vi "Host - INS DVL Data (SubVI).vi"(11 "INS DVL Data":string) -> (3 "INS DVL Data":dbl[](array[numeric]))   [LabVIEW 2021]
panel:
  out "TIME":string
  out "INS Repeater Status":dbl format="%#_15g"
  out "INS System Status LSB":dbl
  out "INS System Status MSB":dbl
  out "INS Algo Status LSB":dbl format="%#_6f"
  out "INS Algo Status MSB":dbl
  out "East speed std":dbl
  out "North speed std":dbl
  out "Vertical speed std":dbl
  out "Longitude std":dbl
  out "Latitude std":dbl
  out "Altitude std":dbl
  out "Roll std":dbl
  out "Heading std":dbl
  out "Pitch std":dbl
  out "SWAY":dbl
  out "SURGE":dbl
  out "HEAVE":dbl
  out "Altitude GPS":dbl format="%#.3f"
  out "GPS Quality Indicator":dbl
  out "GPS Time":dbl format="%#.3f"
  out "Lat GPS":dbl format="%#.8f"
  out "Long GPS":dbl format="%#.8f"
  out "Depth":dbl format="%#.10f"
  out "Depth Time":dbl
  out "East UTM Pos":dbl format="%#.3f"
  out "ALTITUDE":dbl
  out "LAT UTM Zone":string
  out "LONG UTM Zone":string
  out "North UTM Pos":dbl format="%#.3f"
  out "North speed":dbl
  out "East speed":dbl
  out "UP speed":dbl
  out "Longitude":dbl
  out "Latitude":dbl
  out "Altitude":dbl
  out "ROLL":dbl format="%#.10f"
  out "PITCH":dbl
  out "array 7":string[](array[string])
  out "HEADING__2":dbl
  out "array 6":string[](array[string])
  out "HEADING_1":dbl
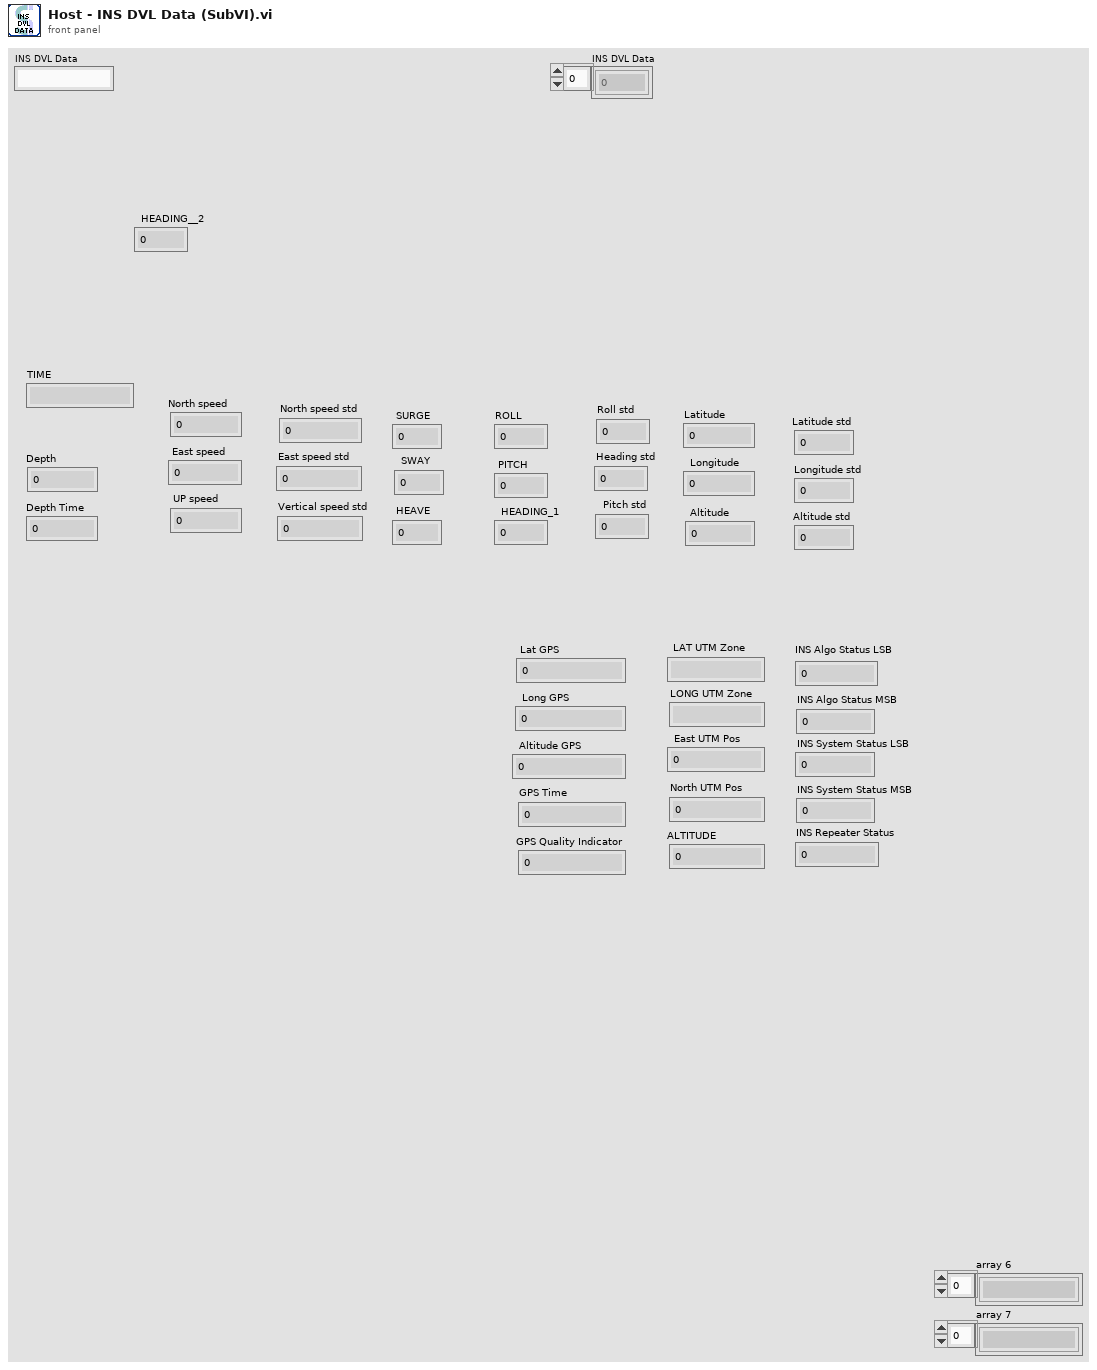
[diagram p1: front panel]
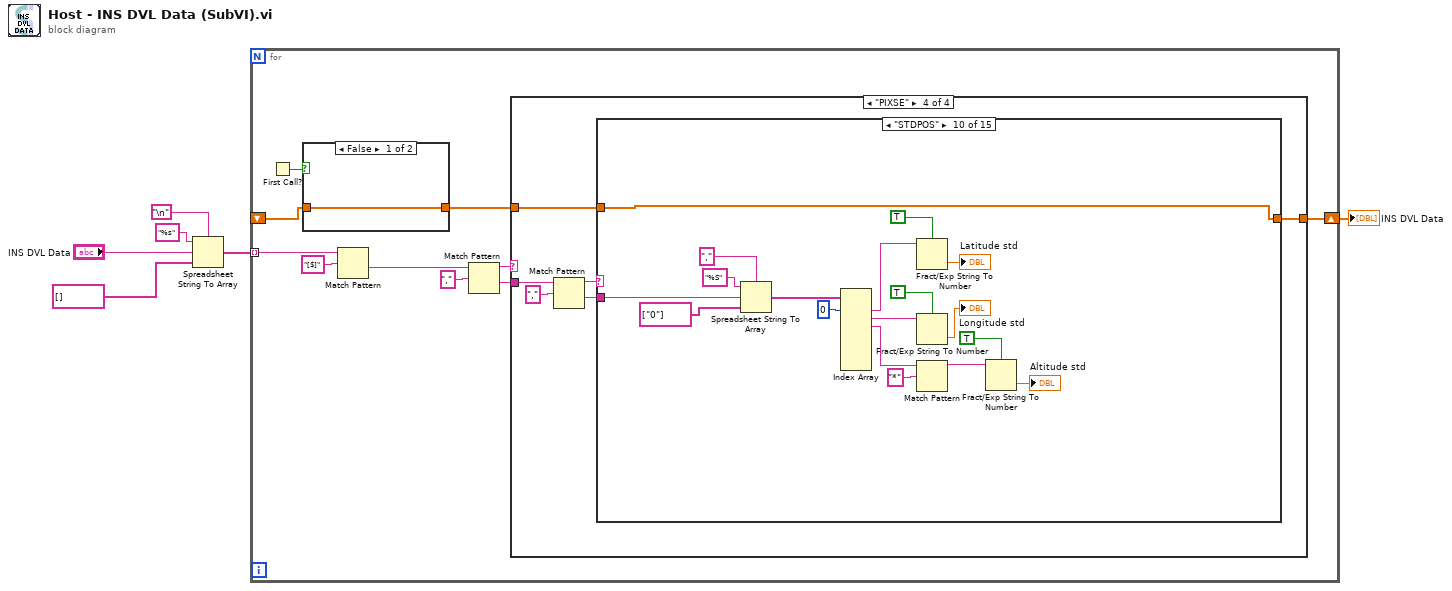
[diagram p0: block diagram]
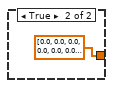
[diagram p2: hidden frame]
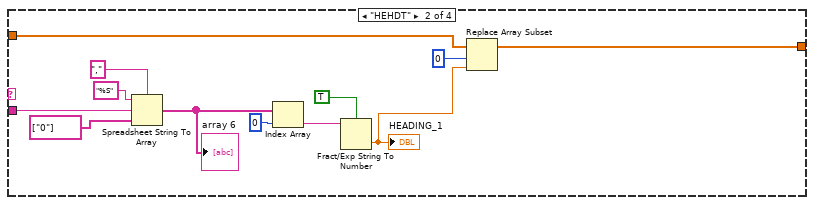
[diagram p4: hidden frame]
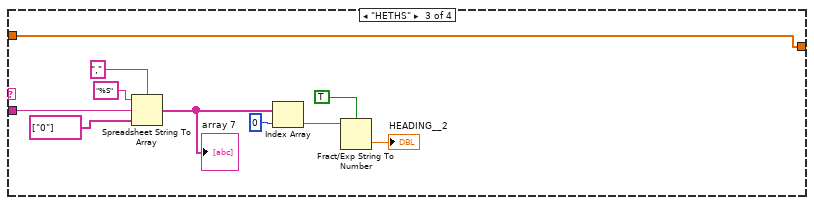
[diagram p5: hidden frame]
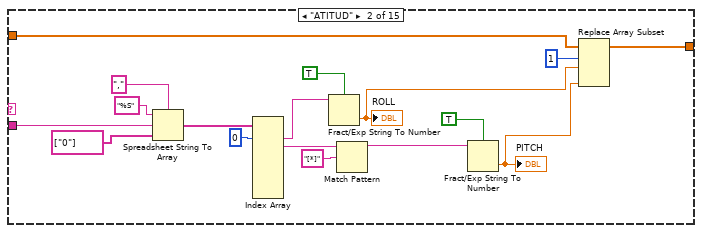
[diagram p7: hidden frame]
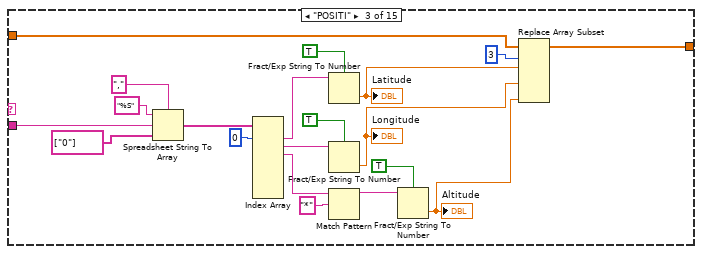
[diagram p8: hidden frame]
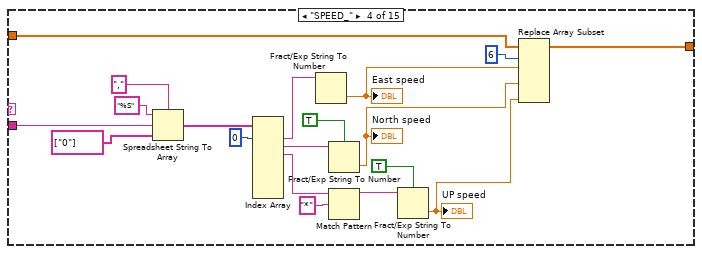
[diagram p9: hidden frame]
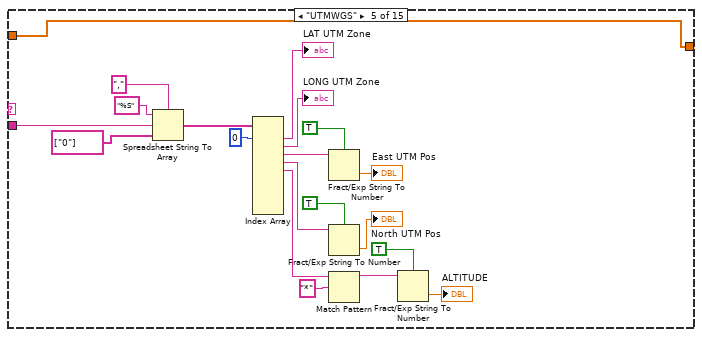
[diagram p10: hidden frame]
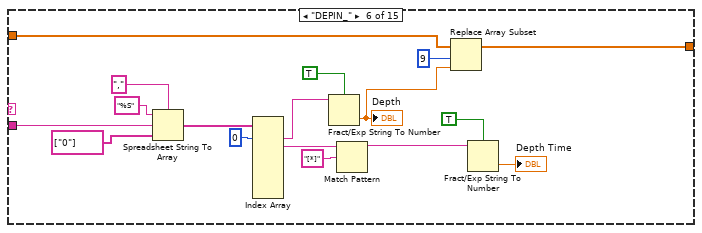
[diagram p11: hidden frame]
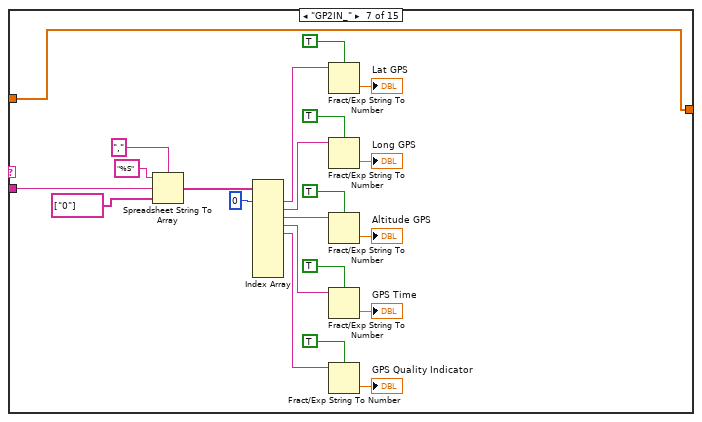
[diagram p12: hidden frame]
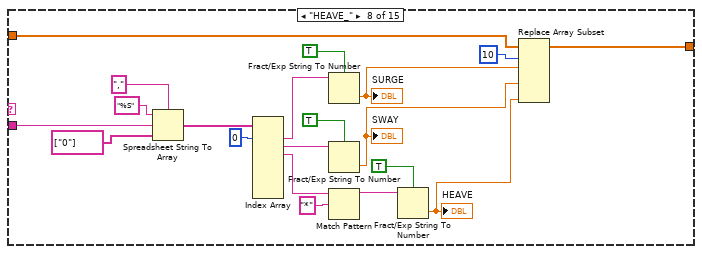
[diagram p13: hidden frame]
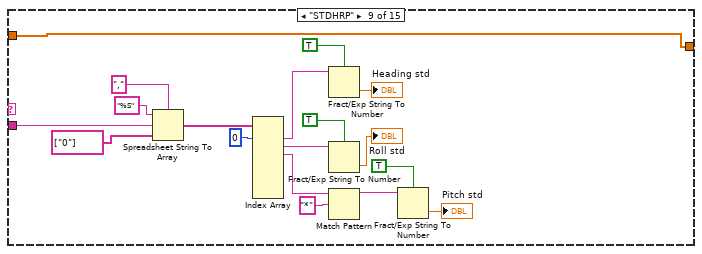
[diagram p14: hidden frame]
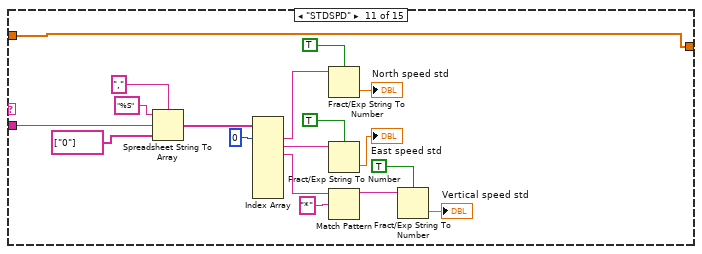
[diagram p15: hidden frame]
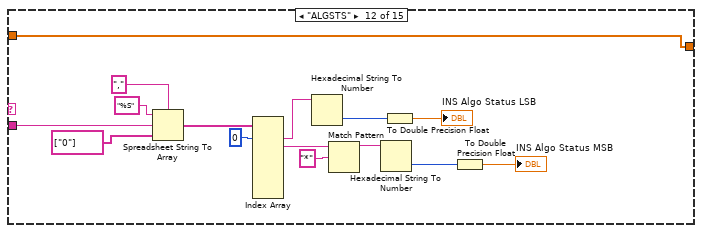
[diagram p16: hidden frame]
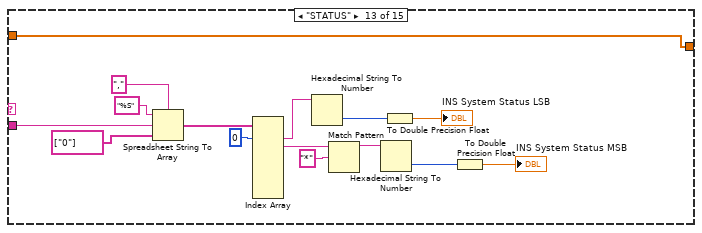
[diagram p17: hidden frame]
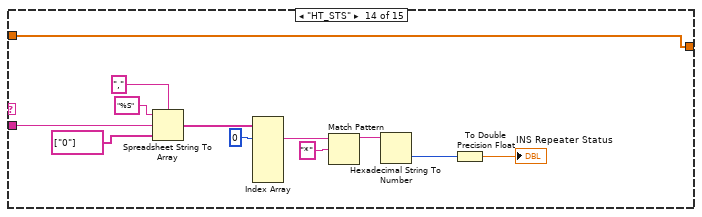
[diagram p18: hidden frame]
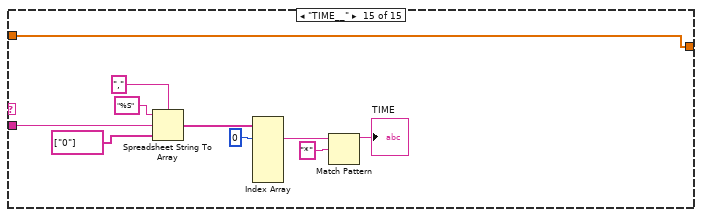
[diagram p19: hidden frame]
diagram:
  n1 = Spreadsheet String To Array(delimiter (Tab)="\n", format string="%s", spreadsheet string="INS DVL Data", array type (2D Dbl)=string[] []) -> (array=w3:string[])
  n2 = for {
    tunnel: w3 -> [w11] mode=indexing
    shift-right: [w10] -> w1
    shift-left: _ -> [w7]
    n3 = First Call?() -> (First Call?: T/F=w9:bool)
    n4 = case shown="False" w9 {
      tunnel: [w17 dbl[] [0.0, 0.0, 0.0, 0.0, 0.0, 0.0, 0.0, 0.0, 0.0, 0.0, 0.0, 0.0, 0.0]] -> w8
      tunnel: w7 -> [w17 _]
      frame False {
      }
      frame True {
      }
    }
    n5 = Match Pattern(string=w11, regular expression="[$]") -> (after substring=w15:string)  [unwired: 1 in, 3 out]
    n6 = Match Pattern(string=w15, regular expression=",") -> (before substring=w13:string, after substring=w12:string)  [unwired: 1 in, 2 out]
    n7 = case shown="\"PIXSE\"" w13 {
      tunnel: w12 -> [_ w28 w38 w47]
      tunnel: w8 -> [w19 w23 w32 w43]
      tunnel: [w19 w22 w32 w42] -> w10
      frame "False", Default {
      }
      frame "HEHDT" {
        n8 = Spreadsheet String To Array(delimiter (Tab)=",", format string="%S", spreadsheet string=w28, array type (2D Dbl)=string[] ["0"]) -> (array=w26:string[])
        "array 6" <- w26
        n9 = Index Array(array=w26, index=0) -> (element=w24:string)
        n10 = Fract/Exp String To Number(use system decimal point (T)=TRUE, string=w24) -> (number=w20:dbl)  [unwired: 2 in, 1 out]
        "HEADING_1" <- w20
        n11 = Replace Array Subset(array=w23, new element=w20, index=0) -> (w22:dbl[])
      }
      frame "HETHS" {
        n12 = Spreadsheet String To Array(delimiter (Tab)=",", format string="%S", spreadsheet string=w38, array type (2D Dbl)=string[] ["0"]) -> (array=w34:string[])
        "array 7" <- w34
        n13 = Index Array(array=w34, index=0) -> (element=w35:string)
        n14 = Fract/Exp String To Number(use system decimal point (T)=TRUE, string=w35) -> (number=→"HEADING__2":dbl)  [unwired: 2 in, 1 out]
      }
      frame "PIXSE" {
        n15 = Match Pattern(string=w47, regular expression=",") -> (before substring=w45:string, after substring=w44:string)  [unwired: 1 in, 2 out]
        n16 = case shown="\"STDPOS\"" w45 {
          tunnel: w44 -> [_ w62 w82 w101 w121 w129 w150 w183 w198 w204 w234 w249 w264 w276 w286]
          tunnel: w43 -> [w48 w53 w70 w90 w105 w127 w142 w168 w184 w202 w220 w238 w253 w268 w280]
          tunnel: [w48 w52 w71 w91 w105 w128 w142 w169 w184 w202 w220 w238 w253 w268 w280] -> w42
          frame "False", Default {
          }
          frame "ATITUD" {
            n17 = Spreadsheet String To Array(delimiter (Tab)=",", format string="%S", spreadsheet string=w62, array type (2D Dbl)=string[] ["0"]) -> (array=w61:string[])
            n18 = Index Array(array=w61, index #1=0 ("index")) -> (element #1=w57:string, element #2=w58:string)  [unwired: 7 in, 6 out]
            n19 = Fract/Exp String To Number(use system decimal point (T)=TRUE, string=w57) -> (number=w50:dbl)  [unwired: 2 in, 1 out]
            "ROLL" <- w50
            n20 = Match Pattern(string=w58, regular expression="[*]") -> (before substring=w55:string)  [unwired: 1 in, 3 out]
            n21 = Fract/Exp String To Number(use system decimal point (T)=TRUE, string=w55) -> (number=w49:dbl)  [unwired: 2 in, 1 out]
            "PITCH" <- w49
            n22 = Replace Array Subset(array=w53, new element #1=w50, index #1=1 ("index"), new element #2=w49) -> (w52:dbl[])  [unwired: 1 in]
          }
          frame "POSITI" {
            n23 = Spreadsheet String To Array(delimiter (Tab)=",", format string="%S", spreadsheet string=w82, array type (2D Dbl)=string[] ["0"]) -> (array=w79:string[])
            n24 = Index Array(array=w79, index #1=0 ("index")) -> (element #1=w81:string, element #2=w72:string, element #3=w74:string)  [unwired: 7 in, 5 out]
            n25 = Fract/Exp String To Number(use system decimal point (T)=TRUE, string=w81) -> (number=w68:dbl)  [unwired: 2 in, 1 out]
            "Latitude" <- w68
            n26 = Fract/Exp String To Number(use system decimal point (T)=TRUE, string=w72) -> (number=w67:dbl)  [unwired: 2 in, 1 out]
            "Longitude" <- w67
            n27 = Match Pattern(string=w74, regular expression="*") -> (before substring=w76:string)  [unwired: 1 in, 3 out]
            n28 = Fract/Exp String To Number(use system decimal point (T)=TRUE, string=w76) -> (number=w66:dbl)  [unwired: 2 in, 1 out]
            "Altitude" <- w66
            n29 = Replace Array Subset(array=w70, new element #1=w68, index #1=3 ("index"), new element #2=w67, new element #3=w66) -> (w71:dbl[])  [unwired: 2 in]
          }
          frame "SPEED_" {
            n30 = Spreadsheet String To Array(delimiter (Tab)=",", format string="%S", spreadsheet string=w101, array type (2D Dbl)=string[] ["0"]) -> (array=w92:string[])
            n31 = Index Array(array=w92, index #1=0 ("index")) -> (element #1=w100:string, element #2=w93:string, element #3=w95:string)  [unwired: 7 in, 5 out]
            n32 = Fract/Exp String To Number(string=w100) -> (number=w88:dbl)  [unwired: 3 in, 1 out]
            "East speed" <- w88
            n33 = Fract/Exp String To Number(use system decimal point (T)=TRUE, string=w93) -> (number=w87:dbl)  [unwired: 2 in, 1 out]
            "North speed" <- w87
            n34 = Match Pattern(string=w95, regular expression="*") -> (before substring=w97:string)  [unwired: 1 in, 3 out]
            n35 = Fract/Exp String To Number(use system decimal point (T)=TRUE, string=w97) -> (number=w86:dbl)  [unwired: 2 in, 1 out]
            "UP speed" <- w86
            n36 = Replace Array Subset(array=w90, new element #1=w88, index #1=6 ("index"), new element #2=w87, new element #3=w86) -> (w91:dbl[])  [unwired: 2 in]
          }
          frame "UTMWGS" {
            n37 = Spreadsheet String To Array(delimiter (Tab)=",", format string="%S", spreadsheet string=w121, array type (2D Dbl)=string[] ["0"]) -> (array=w112:string[])
            n38 = Index Array(array=w112, index #1=0 ("index")) -> (element #1=→"LAT UTM Zone":string, element #2=→"LONG UTM Zone":string, element #3=w111:string, element #4=w106:string, element #5=w109:string)  [unwired: 9 in, 5 out]
            n39 = Fract/Exp String To Number(use system decimal point (T)=TRUE, string=w111) -> (number=→"East UTM Pos":dbl)  [unwired: 2 in, 1 out]
            n40 = Fract/Exp String To Number(use system decimal point (T)=TRUE, string=w106) -> (number=→"North UTM Pos":dbl)  [unwired: 2 in, 1 out]
            n41 = Match Pattern(string=w109, regular expression="*") -> (before substring=w116:string)  [unwired: 1 in, 3 out]
            n42 = Fract/Exp String To Number(use system decimal point (T)=TRUE, string=w116) -> (number=→"ALTITUDE":dbl)  [unwired: 2 in, 1 out]
          }
          frame "DEPIN_" {
            n43 = Spreadsheet String To Array(delimiter (Tab)=",", format string="%S", spreadsheet string=w129, array type (2D Dbl)=string[] ["0"]) -> (array=w138:string[])
            n44 = Index Array(array=w138, index #1=0 ("index")) -> (element #1=w134:string, element #2=w135:string)  [unwired: 7 in, 6 out]
            n45 = Fract/Exp String To Number(use system decimal point (T)=TRUE, string=w134) -> (number=w125:dbl)  [unwired: 2 in, 1 out]
            "Depth" <- w125
            n46 = Match Pattern(string=w135, regular expression="[*]") -> (before substring=w132:string)  [unwired: 1 in, 3 out]
            n47 = Replace Array Subset(array=w127, new element=w125, index=9) -> (w128:dbl[])
            n48 = Fract/Exp String To Number(use system decimal point (T)=TRUE, string=w132) -> (number=→"Depth Time":dbl)  [unwired: 2 in, 1 out]
          }
          frame "GP2IN_" {
            n49 = Spreadsheet String To Array(delimiter (Tab)=",", format string="%S", spreadsheet string=w150, array type (2D Dbl)=string[] ["0"]) -> (array=w155:string[])
            n50 = Index Array(array=w155, index #1=0 ("index")) -> (element #1=w145:string, element #2=w144:string, element #3=w154:string, element #4=w151:string, element #5=w143:string)  [unwired: 9 in, 5 out]
            n51 = Fract/Exp String To Number(use system decimal point (T)=TRUE, string=w145) -> (number=→"Lat GPS":dbl)  [unwired: 2 in, 1 out]
            n52 = Fract/Exp String To Number(use system decimal point (T)=TRUE, string=w144) -> (number=→"Long GPS":dbl)  [unwired: 2 in, 1 out]
            n53 = Fract/Exp String To Number(use system decimal point (T)=TRUE, string=w154) -> (number=→"Altitude GPS":dbl)  [unwired: 2 in, 1 out]
            n54 = Fract/Exp String To Number(use system decimal point (T)=TRUE, string=w151) -> (number=→"GPS Time":dbl)  [unwired: 2 in, 1 out]
            n55 = Fract/Exp String To Number(use system decimal point (T)=TRUE, string=w143) -> (number=→"GPS Quality Indicator":dbl)  [unwired: 2 in, 1 out]
          }
          frame "HEAVE_" {
            n56 = Spreadsheet String To Array(delimiter (Tab)=",", format string="%S", spreadsheet string=w183, array type (2D Dbl)=string[] ["0"]) -> (array=w171:string[])
            n57 = Index Array(array=w171, index #1=0 ("index")) -> (element #1=w176:string, element #2=w179:string, element #3=w178:string)  [unwired: 7 in, 5 out]
            n58 = Fract/Exp String To Number(use system decimal point (T)=TRUE, string=w176) -> (number=w166:dbl)  [unwired: 2 in, 1 out]
            "SURGE" <- w166
            n59 = Fract/Exp String To Number(use system decimal point (T)=TRUE, string=w179) -> (number=w165:dbl)  [unwired: 2 in, 1 out]
            "SWAY" <- w165
            n60 = Match Pattern(string=w178, regular expression="*") -> (before substring=w177:string)  [unwired: 1 in, 3 out]
            n61 = Fract/Exp String To Number(use system decimal point (T)=TRUE, string=w177) -> (number=w164:dbl)  [unwired: 2 in, 1 out]
            "HEAVE" <- w164
            n62 = Replace Array Subset(array=w168, new element #1=w166, index #1=10 ("index"), new element #2=w165, new element #3=w164) -> (w169:dbl[])  [unwired: 2 in]
          }
          frame "STDHRP" {
            n63 = Spreadsheet String To Array(delimiter (Tab)=",", format string="%S", spreadsheet string=w198, array type (2D Dbl)=string[] ["0"]) -> (array=w186:string[])
            n64 = Index Array(array=w186, index #1=0 ("index")) -> (element #1=w197:string, element #2=w188:string, element #3=w190:string)  [unwired: 7 in, 5 out]
            n65 = Fract/Exp String To Number(use system decimal point (T)=TRUE, string=w197) -> (number=→"Heading std":dbl)  [unwired: 2 in, 1 out]
            n66 = Fract/Exp String To Number(use system decimal point (T)=TRUE, string=w188) -> (number=→"Roll std":dbl)  [unwired: 2 in, 1 out]
            n67 = Match Pattern(string=w190, regular expression="*") -> (before substring=w193:string)  [unwired: 1 in, 3 out]
            n68 = Fract/Exp String To Number(use system decimal point (T)=TRUE, string=w193) -> (number=→"Pitch std":dbl)  [unwired: 2 in, 1 out]
          }
          frame "STDPOS" {
            n69 = Spreadsheet String To Array(delimiter (Tab)=",", format string="%S", spreadsheet string=w204, array type (2D Dbl)=string[] ["0"]) -> (array=w219:string[])
            n70 = Index Array(array=w219, index #1=0 ("index")) -> (element #1=w212:string, element #2=w218:string, element #3=w217:string)  [unwired: 7 in, 5 out]
            n71 = Fract/Exp String To Number(use system decimal point (T)=TRUE, string=w212) -> (number=→"Latitude std":dbl)  [unwired: 2 in, 1 out]
            n72 = Fract/Exp String To Number(use system decimal point (T)=TRUE, string=w218) -> (number=→"Longitude std":dbl)  [unwired: 2 in, 1 out]
            n73 = Match Pattern(string=w217, regular expression="*") -> (before substring=w215:string)  [unwired: 1 in, 3 out]
            n74 = Fract/Exp String To Number(use system decimal point (T)=TRUE, string=w215) -> (number=→"Altitude std":dbl)  [unwired: 2 in, 1 out]
          }
          frame "STDSPD" {
            n75 = Spreadsheet String To Array(delimiter (Tab)=",", format string="%S", spreadsheet string=w234, array type (2D Dbl)=string[] ["0"]) -> (array=w222:string[])
            n76 = Index Array(array=w222, index #1=0 ("index")) -> (element #1=w233:string, element #2=w227:string, element #3=w228:string)  [unwired: 7 in, 5 out]
            n77 = Fract/Exp String To Number(use system decimal point (T)=TRUE, string=w233) -> (number=→"North speed std":dbl)  [unwired: 2 in, 1 out]
            n78 = Fract/Exp String To Number(use system decimal point (T)=TRUE, string=w227) -> (number=→"East speed std":dbl)  [unwired: 2 in, 1 out]
            n79 = Match Pattern(string=w228, regular expression="*") -> (before substring=w230:string)  [unwired: 1 in, 3 out]
            n80 = Fract/Exp String To Number(use system decimal point (T)=TRUE, string=w230) -> (number=→"Vertical speed std":dbl)  [unwired: 2 in, 1 out]
          }
          frame "ALGSTS" {
            n81 = Spreadsheet String To Array(delimiter (Tab)=",", format string="%S", spreadsheet string=w249, array type (2D Dbl)=string[] ["0"]) -> (array=w246:string[])
            n82 = Index Array(array=w246, index #1=0 ("index")) -> (element #1=w245:string, element #2=w244:string)  [unwired: 7 in, 6 out]
            n83 = Hexadecimal String To Number(string=w245) -> (number=w242:u32)  [unwired: 2 in, 1 out]
            n84 = Match Pattern(string=w244, regular expression="*") -> (before substring=w243:string)  [unwired: 1 in, 3 out]
            n85 = Hexadecimal String To Number(string=w243) -> (number=w240:u32)  [unwired: 2 in, 1 out]
            n86 = To Double Precision Float(number=w242) -> (double precision float=→"INS Algo Status LSB":dbl)
            n87 = To Double Precision Float(number=w240) -> (double precision float=→"INS Algo Status MSB":dbl)
          }
          frame "STATUS" {
            n88 = Spreadsheet String To Array(delimiter (Tab)=",", format string="%S", spreadsheet string=w264, array type (2D Dbl)=string[] ["0"]) -> (array=w260:string[])
            n89 = Index Array(array=w260, index #1=0 ("index")) -> (element #1=w262:string, element #2=w261:string)  [unwired: 7 in, 6 out]
            n90 = Hexadecimal String To Number(string=w262) -> (number=w258:u32)  [unwired: 2 in, 1 out]
            n91 = Match Pattern(string=w261, regular expression="*") -> (before substring=w256:string)  [unwired: 1 in, 3 out]
            n92 = Hexadecimal String To Number(string=w256) -> (number=w255:u32)  [unwired: 2 in, 1 out]
            n93 = To Double Precision Float(number=w258) -> (double precision float=→"INS System Status LSB":dbl)
            n94 = To Double Precision Float(number=w255) -> (double precision float=→"INS System Status MSB":dbl)
          }
          frame "HT_STS" {
            n95 = Spreadsheet String To Array(delimiter (Tab)=",", format string="%S", spreadsheet string=w276, array type (2D Dbl)=string[] ["0"]) -> (array=w275:string[])
            n96 = Index Array(array=w275, index #1=0 ("index")) -> (element #1=w271:string)  [unwired: 5 in, 5 out]
            n97 = Match Pattern(string=w271, regular expression="*") -> (before substring=w273:string)  [unwired: 1 in, 3 out]
            n98 = Hexadecimal String To Number(string=w273) -> (number=w270:u32)  [unwired: 2 in, 1 out]
            n99 = To Double Precision Float(number=w270) -> (double precision float=→"INS Repeater Status":dbl)
          }
          frame "TIME__" {
            n100 = Spreadsheet String To Array(delimiter (Tab)=",", format string="%S", spreadsheet string=w286, array type (2D Dbl)=string[] ["0"]) -> (array=w282:string[])
            n101 = Index Array(array=w282, index #1=0 ("index")) -> (element #1=w285:string)  [unwired: 5 in, 5 out]
            n102 = Match Pattern(string=w285, regular expression="*") -> (before substring=→"TIME":string)  [unwired: 1 in, 3 out]
          }
        }
      }
    }
  }
  "INS DVL Data" <- w1
